vi "LJUD UE9RAW Reset.vi"(5 "Comm Settings":T1={"Open LabJack "=TRUE, "Use USB"=TRUE, "IP Address"="192.168.1.209", "PortA"=52360, "PortB"=0}, 8 "error in (no error)":errorcluster, 10 "Soft Reset Only":bool, 11 "Handle In":i32) -> (0 "error out":errorcluster, 3 "Handle Out":i32)   [LabVIEW 2021]
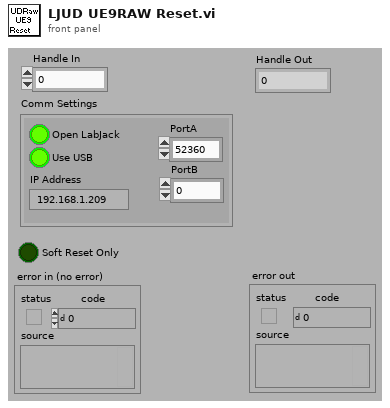
[diagram p1: front panel]
types:
  T1 = cluster{"Open LabJack ":bool, "Use USB":bool, "IP Address":string, "PortA":u16, "PortB":u16}
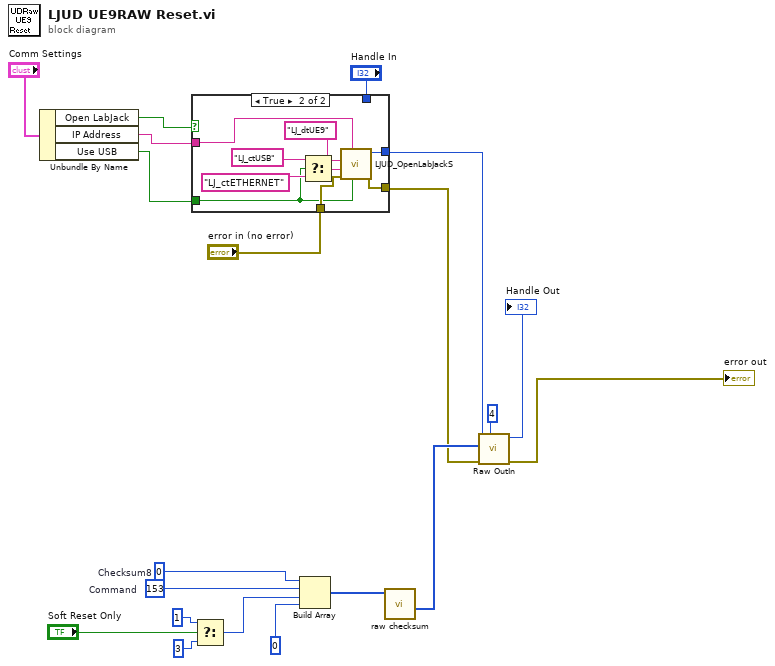
[diagram p0: block diagram]
diagram:
  w18 = u8 0  # Checksum8
  w20 = u8 153  # Command
  n1 = Unbundle By Name("Comm Settings") -> ("Open LabJack"=w7:bool, "IP Address"=w6:string, "Use USB"=w5:bool)
  n2 = case shown="True" w7 {
    tunnel: w6 -> [_ w25]
    tunnel: "error in (no error)" -> [w22 w29]
    tunnel: [w22 w28] -> w3
    tunnel: [w21 w26] -> w2
    tunnel: w5 -> [_ w27]
    tunnel: "Handle In" -> [w21 _]
    frame False {
    }
    frame True {
      n3 = Select(t="LJ_ctUSB" ("ConnectionType"), s=w27, f="LJ_ctETHERNET" ("ConnectionType")) -> (s? t:f=w23:string)
      n4 = call "LJUD_OpenLabJackS.vi"("FirstFound"=w27, "Address"=w25, "error in"=w29, "ConnectionType"=w23, "DeviceType"="LJ_dtUE9") -> ("error out"=w28:errorcluster, "Handle"=w26:i32)  [unwired: 4 in, 1 out]
    }
  }
  n5 = Select(t=u8 1 ("Input Element"), s="Soft Reset Only", f=u8 3 ("Input Element")) -> (s? t:f=w11:u8)
  n6 = Build Array(w18, w20, w11, u8 0 ("Input Element")) -> (w19:u8[])
  n7 = call "raw checksum.vi"("Array"=w19) -> ("Array Output"=w17:u8[])  [unwired: 3 in, 7 out]
  n8 = call "Raw OutIn.vi"("# of bytes to read in"=4 ("# of bytes to read"), "error in"=w3, "Raw Out"=w17, "Handle In"=w2) -> ("error out"=→"error out":errorcluster, "Handle Out"=→"Handle Out":i32)  [unwired: 4 in, 2 out]
